vi "Auto Elevator Logic.vi"(8 "Has Trashcan?":bool, 10 "Elevator Sensors In":T7, 11 "Command":T3={"Command"=enum."Idle", "Manual Motor Out"=0.0, "Manual Eject Piston"=FALSE, "Mode"=enum."Manual", "Override Limits"=FALSE, "Manual Stabilizer"=FALSE, "Manual Finger"=FALSE, "Store Trashcan?"=FALSE, "Hold Low?"=FALSE, "Idle Mode"=enum."Load Can", "HP Load"=FALSE, "Unstick"=FALSE, "Raw Height Set"=0.0, "Force Store"=FALSE}) -> (0 "Trashcan Delta":i32, 1 "Tote Delta":i16, 2 "Elevator Actuators Out":T8, 3 "Auto Elevator Indicators":T1, 4 "Clear Stack Count":bool)   [LabVIEW 2014]
uses:
  Elevator Actuators.ctl
  Elevator Sensors.ctl
  Elevator Control Command.ctl
  Elevator Command.ctl
  Common Code/Elevator Mode.ctl
  Common Code/Elevator Idle Mode.ctl
  Common Code/Auto Elevator Indicators.ctl
  Common Code/Elevator State.ctl
  <vilib>/Rock Robotics/WPI/DriverStation/WPI_DriverStationRobotMode2.ctl
  Common Code/Change Detect Int.vi
  Robot Global Data.vi
panel:
  in  "# Totes Loading":i32
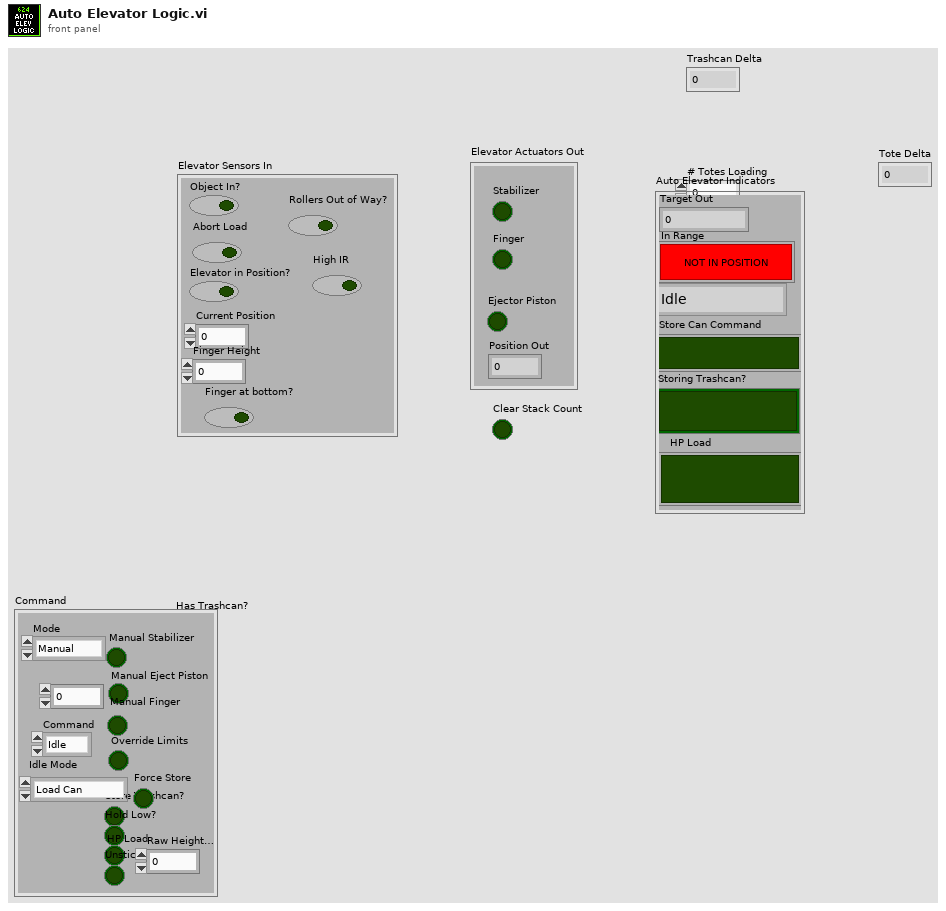
[diagram p1: front panel]
types:
  T1 = typedef "Auto Elevator Indicators.ctl" = cluster{"Target Out":dbl, "Storing Trashcan?":bool, "State":T2, "In Range":bool, "Store Can Command":bool, "HP Load":bool}
  T2 = typedef "Elevator State.ctl" = enum16{"Idle", "Goto Load Position", "Wait for Load", "Load Drop", "Load Lift", "Drop Stack", "Goto Eject Position", "Eject ", "Raise Trashcan", "Open Stabilizer", "Untip Drop", "Untip Wait", "Untip Lift", "Abort Load", "HP Load Wait", "HP Load Drop", "HP Load Lift", "HP Load Abort", "Close Stabilizer", "HP Load Unfinish", "HP Load Score", "HP Load Finish", "HP Goto Finish Down", "HP Goto Finish Up", "Full"}
  T3 = typedef "Elevator Control Command.ctl" = cluster{"Command":T4, "Manual Motor Out":dbl, "Manual Eject Piston":bool, "Mode":T5, "Override Limits":bool, "Manual Stabilizer":bool, "Manual Finger":bool, "Store Trashcan?":bool, "Hold Low?":bool, "Idle Mode":T6, "HP Load":bool, "Unstick":bool, "Raw Height Set":dbl, "Force Store":bool}
  T4 = typedef "Elevator Command.ctl" = enum16{"Idle", "Load 1", "Load 2", "Load 3", "Drop Stack", "Eject Stack", "Untip Trashcan", "Load Trashcan", "HP Load", "HP Score"}
  T5 = typedef "Elevator Mode.ctl" = enum16{"Manual", "Safe", "Auto"}
  T6 = typedef "Elevator Idle Mode.ctl" = enum16{"Load 1", "Load 2", "Load 3", "Load Can", "Untip Can", "Step Load", "Drop Stack", "Raw Height"}
  T7 = typedef "Elevator Sensors.ctl" = cluster{"Object In?":bool, "Elevator in Position?":bool, "Current Position":dbl, "Abort Load":bool, "Finger Height":dbl, "Finger at bottom?":bool, "Rollers Out of Way?":bool, "High IR":bool}
  T8 = typedef "Elevator Actuators.ctl" = cluster{"Ejector Piston":bool, "Finger":bool, "Stabilizer":bool, "Position Out":dbl}
  T9 = typedef "WPI_DriverStationRobotMode2.ctl" = enum16{"Autonomous Disabled", "Autonomous Enabled", "Teleop Disabled", "Teleop Enabled", "Disconnected", "Finish", "Test Disabled", "Test Enabled", "Emergency Stopped"}
  T10 = typedef "Dashboard Control Data.ctl" = cluster{"Cam Exposure":dbl, "Go to angle":dbl, "Steer PID Gains":cluster{"proportional gain (Kc)":dbl, "integral time (Ti, min)":dbl, "derivative time (Td, min)":dbl}, "Steer PID output Range":cluster{"output high":dbl, "output low":dbl}, "Pressure m \nValue":dbl, "Pressure b \nValue":dbl, "Roller Command Cluster ":T11, "Elevator":T12, "Encoder Control":T14, "Auton Settings":cluster{"Drive Dist Window Size":dbl}, "Drivetrain Settings":T15, "Lance":T16}
  T11 = typedef "Roller Control.ctl" = cluster{"Intake Speed":dbl, "Turn In Speed":dbl, "Unload Speed":dbl, "Turn Out Speed":dbl, "Ping Align Tolerance":dbl, "Tote Range Threshold":dbl, "Right Pot 0":dbl, "Pot Threshold":dbl, "Left Pot 0":dbl, "Right Pot Scale":dbl, "Left Pot Scale":dbl, "Min Elevator Height":dbl, "Eject Time":dbl, "Eject US Threshold":dbl, "Anti-Twitch Time":u32, "Ping Caring Threshold":dbl, "Pot Diff Threshold":dbl, "Pinch Sustain":u32, "Absorb Give Up Threshold":dbl, "Untip In Threshold":dbl, "Untip Grab Range":dbl, "Ultrasonic Hold Time":u32, "Landscape Absorb Time":u32, "Pot Use Wait Time":u32, "Can Turn Stop Range":dbl, "HP Load Speed":dbl, "Stick Multiplier":dbl}
  T12 = typedef "Elevator DB Control.ctl" = cluster{"PID Output Range":cluster{"output high":dbl, "output low":dbl}, "PID gains":cluster{"proportional gain (Kc)":dbl, "integral time (Ti, min)":dbl, "derivative time (Td, min)":dbl}, "Height Tolerance":sgl, " Encoder Constant":dbl, "Eject Time":sgl, "Zeroing Speed":sgl, "Presets":T13, "Ping Detect Threshold":sgl, "Trashcan Detect Threshold":sgl, "Zero Filter Time":dbl, "Stabilizer Open Time":dbl, "Zero Creep Speed":dbl, "Max Current":dbl, "Current Trip Time":dbl, "Abort Pitch":dbl, "Finger m":dbl, "Finger b":dbl, "Finger max ":dbl, "Finger Stabilizer":dbl, "Finger Store":dbl, "Finger Stop Store":dbl, "Stabilizer Close Time":dbl, "Finger min":dbl, "Unstick gain":dbl, "Full Detect Max":dbl}
  T13 = typedef "Elevator Presets.ctl" = cluster{"Pickup 2 w/ Tote":sgl, "Pickup 2 w/ Trashcan":sgl, "Pickup 3 w/ Tote":sgl, "Pickup 3 w/ Trashcan":sgl, "Bottom":sgl, "Pickup 1 w/ Tote":sgl, "Pickup Trashcan":sgl, "Pickup 1 w/ Trashcan":sgl, "Eject":sgl, "Hold Low":sgl, "Step add height":sgl, "Untip Lift":dbl, "Drop Stack":dbl, "HP Load Hold":dbl, "HP Load Drop":dbl, "HP Load Hold Can":dbl, "Store can max":dbl, "HP Drag Score":dbl, "HP Drag Finish":dbl, "Finger trashcan avoid":dbl, "Full":dbl}
  T14 = typedef "Encoder Control.ctl" = cluster{"Left Tick Constant":dbl, "Right Tick Constant":dbl, "Center Tick Constant":dbl, "Reset?":bool, "Y Dist":cluster{"PID gains":cluster{"proportional gain (Kc)":dbl, "integral time (Ti, min)":dbl, "derivative time (Td, min)":dbl}}, "X Dist":cluster{"PID gains":cluster{"proportional gain (Kc)":dbl, "integral time (Ti, min)":dbl, "derivative time (Td, min)":dbl}}, "Y Stop Thresh":dbl, "Y Stop Speed":dbl, "X Stop Thresh":dbl, "X Stop Speed":dbl}
  T15 = typedef "Drivetrain Settings.ctl" = cluster{"Gyro Tolerance":sgl, "Strafe Correct max steer":sgl, "Strafe Timer Wait":sgl, "Throttle Ramp (ms)":sgl, "Strafe Ramp (ms)":sgl, "Angular rate compensation":bool, "Throttle to Rate Scale":sgl, "Rate compensation gain":sgl, "Creep Steer":sgl, "Creep Throttle":sgl}
  T16 = typedef "Pike DB Controls.ctl" = cluster{"Down Speed":dbl, "Up Speed":dbl, "Max Down Time":dbl, "Max Up Time":dbl, "Current Limit":dbl}
  T17 = typedef "Roller Indicators.ctl" = cluster{"Rollers Closed?":bool, "Roller Mode":T18, "Auto Roller State":T19, "Tote Inside?":bool, "Intake State":T20, "Left Ping Dist":sgl, "Right Ping Dist":sgl, "Potentiometer Cluster":T21, "PING Decision":T20, "Left Arm Closed?":bool, "Portrait?":bool, "Right Arm Closed?":bool, "Left Out":sgl, "Right Out":sgl, "Left Current":sgl, "Right Current":sgl, "Tote Load Complete?":bool, "Untip Complete?":bool, "Untip State":T22, "Roller Safety Open":bool}
  T18 = typedef "Roller Mode Enum.ctl" = enum16{"Manual", "Safe", "Auto"}
  T19 = typedef "Auto Roller Commands.ctl" = enum16{"Drag Tote", "Grab Tote", "Idle", "Eject Tote", "Untip Can", "Grab Can"}
  T20 = typedef "Inner Roller States.ctl" = enum16{"Turn Tote Portrait", "Acquire Tote", "Absorb Tote", "Turn Tote Right", "Turn Tote Left", "Acquire Can", "Absorb Can", "Turn Can", "Hold Tote"}
  T21 = typedef "Pot Data.ctl" = cluster{"Left Pot Zero":sgl, "Right Pot Zero":sgl, "Left Potentiometer":sgl, "Right Potentiometer":sgl, "Left Pot Non Zero":sgl, "Right Pot Non Zero":sgl}
  T22 = typedef "Untip Can States.ctl" = enum16{"Release Can", "Catch Can", "Idle"}
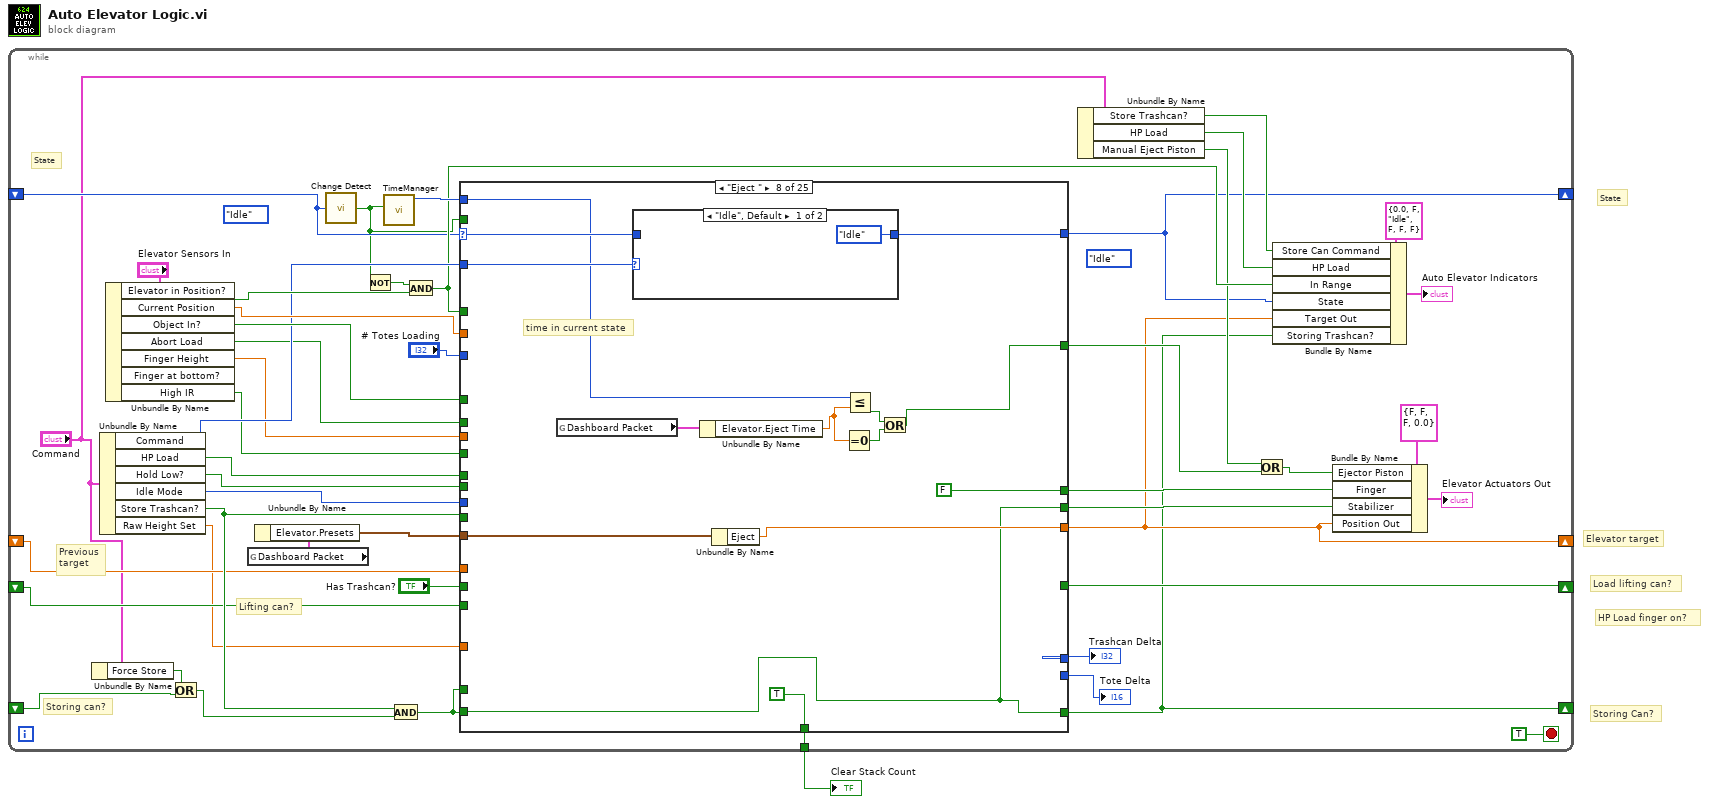
[diagram p0: block diagram]
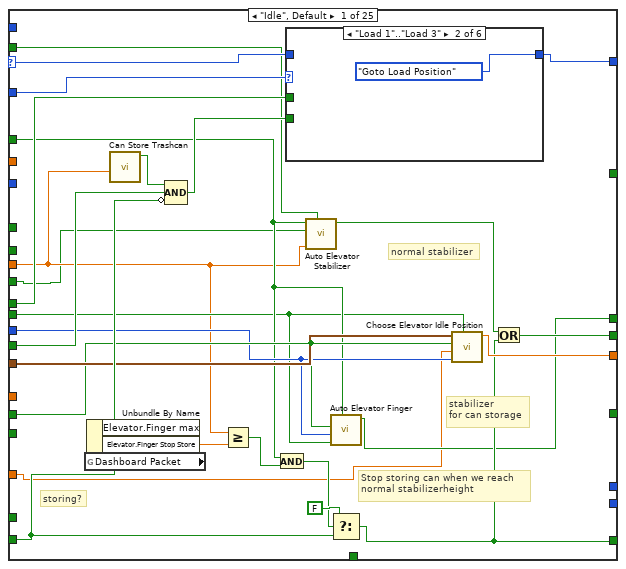
[diagram p2: hidden frame]
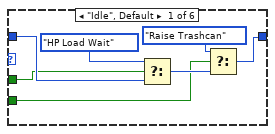
[diagram p3: hidden frame]
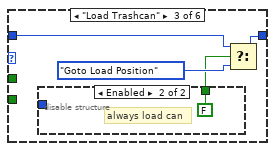
[diagram p4: hidden frame]
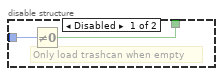
[diagram p5: hidden frame]
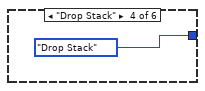
[diagram p6: hidden frame]
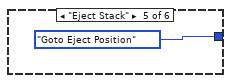
[diagram p7: hidden frame]
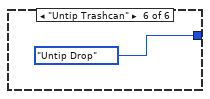
[diagram p8: hidden frame]
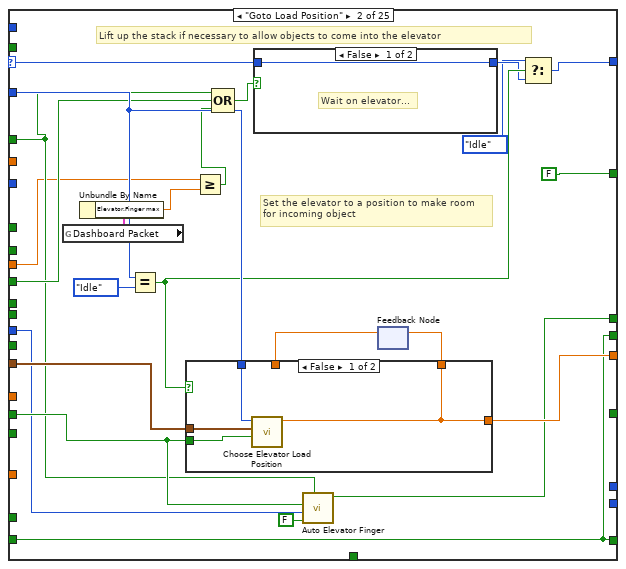
[diagram p9: hidden frame]
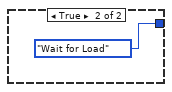
[diagram p11: hidden frame]
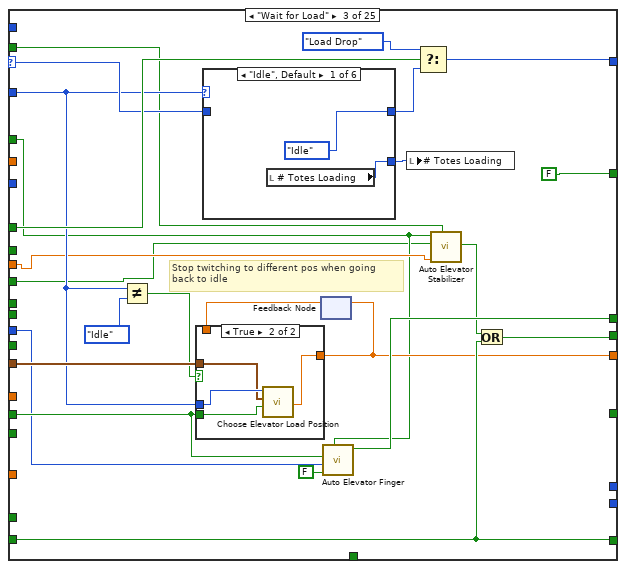
[diagram p12: hidden frame]
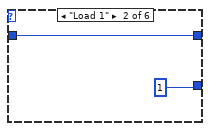
[diagram p13: hidden frame]
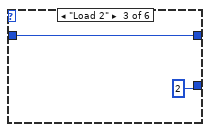
[diagram p14: hidden frame]
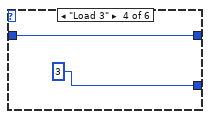
[diagram p15: hidden frame]
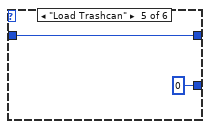
[diagram p16: hidden frame]
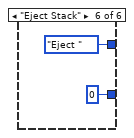
[diagram p17: hidden frame]
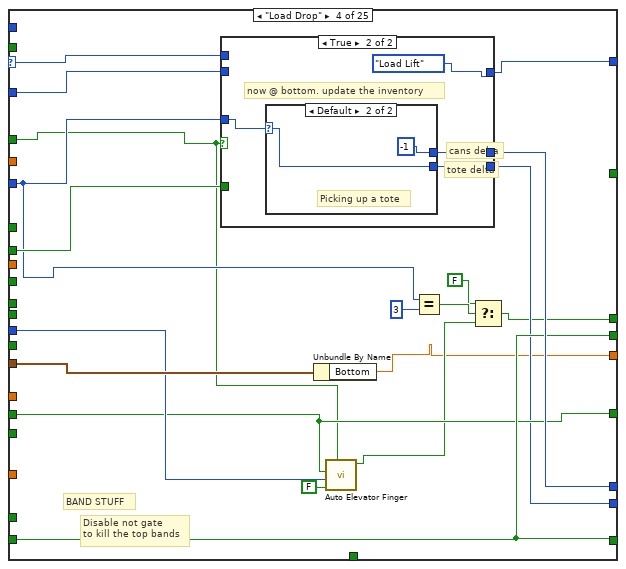
[diagram p19: hidden frame]
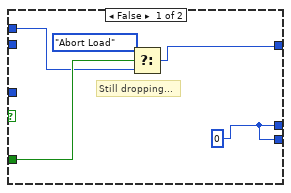
[diagram p20: hidden frame]
diagram:
  # "State"
  # "Storing Can?"
  # "HP Load finger on?"
  # "Load lifting can?"
  # "Elevator target"
  n1 = while {
    tunnel: [w39] -> w1
    shift-right: [w18] -> _
    shift-left: _ -> [w17]
    shift-right: [w16] -> _
    shift-left: _ -> [w15]
    shift-right: [w14] -> _
    shift-left: _ -> [w4]
    shift-right: [w8] -> _
    shift-left: _ -> [w13]
    stop <- TRUE stop-if-true
    (unwired) Elevator_State."Idle" ("f")
    (unwired) Elevator_State."Idle" ("f")
    # "Storing can?"
    # "State"
    # "Lifting can?"
    # "Previous\ntarget"
    n2 = Unbundle By Name("Command") -> ("Force Store"=w3:bool)
    n3 = Unbundle By Name("Command") -> ("Command"=w36:T4, "HP Load"=w28:bool, "Hold Low?"=w31:bool, "Idle Mode"=w30:T6, "Store Trashcan?"=w35:bool, "Raw Height Set"=w6:dbl)
    n4 = Unbundle By Name("Elevator Sensors In") -> ("Elevator in Position?"=w47:bool, "Current Position"=w45:dbl, "Object In?"=w46:bool, "Abort Load"=w29:bool, "Finger Height"=w22:dbl, "High IR"=w7:bool)  [unwired: 1 out]
    n5 = Or(x=w3, y=w4) -> (x .or. y?=w2:bool)
    n6 = global read "Robot Global Data.vi" "Dashboard Packet"() -> (w12:T10)
    n7 = Unbundle By Name(w12) -> ("Elevator.Presets"=w38:T13)
    n8 = call-poly "Change Detect.vi"("In"=w13) -> ("Changed?"=w9:bool)
    n9 = Not(x=w9) -> (.not. x?=w49:bool)
    n10 = call "TimeManager.vi"("Reset?"=w9) -> ("Time Since Reset"=w37:u32)  [unwired: 9 in, 1 out]
    n11 = And(x=w35, y=w2) -> (x .and. y?=w10:bool)
    n12 = And(x=w49, y=w47) -> (x .and. y?=w32:bool)
    n13 = case shown="\"Eject \"" w13 {
      selector: w13 -> [w59 w116 w146 w182 w231 w254 w271 w290 w304 w332 w351 w366 w376 w398 w410 w460 w477 w487 w501 w507 w516 w528 w540 w556 w570]
      tunnel: [_ FALSE ("Ejector Piston") FALSE ("Ejector Piston") _ FALSE ("Ejector Piston") FALSE ("Ejector Piston") FALSE ("Ejector Piston") w283 FALSE ("Ejector Piston") FALSE ("Ejector Piston") w355 w369 w379 _ _ _ _ _ _ _ _ _ _ _ _] -> w25
      tunnel: w38 -> [w65 w115 w143 w185 w218 w257 w275 w293 _ w331 w357 w371 w381 w390 w409 w462 w464 w493 _ _ w522 _ w545 w567 w577]
      tunnel: [w75 w118 w139 w168 w228 w256 w274 w292 w299 w323 w356 w370 w380 w396 w419 w461 w463 w481 w496 w513 w521 w525 w544 w566 w576] -> w18
      tunnel: w45 -> [_ _ _ _ w206 _ _ _ _ w322 _ _ _ _ w408 _ _ _ _ _ _ w525 _ _ _]
      tunnel: w46 -> [_ _ w148 _ _ w253 _ _ _ _ _ _ _ _ _ _ _ _ _ _ _ _ _ _ _]
      tunnel: w36 -> [w76 w112 w137 w183 w235 w255 w272 w291 w312 w336 w354 w364 w374 w394 w412 _ _ w492 _ _ w518 w530 w541 w557 w572]
      tunnel: w32 -> [w56 w100 w130 w167 w204 w248 w267 _ _ w329 w348 _ _ w386 _ w459 w475 w489 _ _ _ _ w539 w561 _]
      tunnel: "# Totes Loading" -> [_ _ _ w175 _ _ _ _ _ _ _ _ _ _ _ _ _ _ _ _ _ _ _ _ _]
      tunnel: "Has Trashcan?" -> [w62 w105 w132 w178 w226 w250 w269 _ _ _ _ _ _ w388 w405 w451 _ w478 _ _ _ _ _ _ _]
      tunnel: [_ _ _ w184 _ _ _ _ _ w341 _ _ _ _ _ _ -1 ("f") _ _ _ _ _ _ _ _] -> w41
      tunnel: [w57 w113 w140 w170 w224 w245 w270 FALSE TRUE TRUE w355 w369 w379 w403 w406 w450 TRUE ("Boolean") w479 TRUE ("Boolean") TRUE ("Boolean") w520 w527 TRUE ("Boolean") TRUE ("Boolean") TRUE ("Boolean")] -> w21
      tunnel: [w72 w114 w141 w181 w220 w245 w264 w281 FALSE FALSE w355 w369 w379 w402 w413 w452 w469 FALSE TRUE ("Close stabilizer") FALSE ("Boolean") w520 w527 FALSE ("Boolean") w548 TRUE ("t")] -> w20
      tunnel: [_ _ _ _ _ w252 _ TRUE _ _ _ _ _ _ _ _ _ _ _ _ _ _ _ _ _] -> w39
      tunnel: w37 -> [_ _ _ _ _ _ _ w287 w307 _ _ _ _ _ _ _ _ _ w504 w508 _ _ _ _ _]
      tunnel: [w71 w114 w142 w181 w222 FALSE w264 w281 FALSE ("x >= y?") w327 FALSE ("x >= y?") FALSE ("x >= y?") FALSE ("x >= y?") w401 w413 w452 w469 FALSE ("x >= y?") TRUE ("x >= y?") FALSE ("x >= y?") FALSE ("t") FALSE ("t") FALSE ("t") w548 FALSE ("t")] -> w14
      tunnel: w10 -> [w69 w114 w142 w181 w222 _ w264 w281 _ _ _ _ _ w401 w415 w452 w471 _ _ _ _ _ _ w554 _]
      tunnel: w35 -> [w70 _ _ _ _ _ _ _ w313 w337 _ _ _ _ _ _ _ _ _ _ _ _ _ _ _]
      tunnel: w31 -> [w55 _ _ _ w229 w247 _ _ _ _ _ _ _ _ _ _ _ _ _ _ _ _ _ _ _]
      tunnel: w30 -> [w61 w104 w131 w179 w227 _ w268 _ _ _ _ _ _ w387 _ _ _ _ _ _ _ _ _ _ _]
      tunnel: w29 -> [_ _ _ w180 _ _ _ _ _ _ _ _ _ _ _ w456 _ _ _ _ _ _ _ _ _]
      tunnel: w28 -> [w58 _ _ _ _ _ _ _ _ _ _ _ _ _ w411 _ _ _ _ _ _ _ _ _ _]
      tunnel: w22 -> [w53 w98 w133 _ w214 _ _ _ w301 w321 _ _ _ w389 w404 _ w473 _ _ _ _ _ _ w553 _]
      tunnel: [_ _ _ w178 w216 _ _ _ _ _ _ _ _ _ _ _ _ _ _ _ _ _ _ _ _] -> w16
      tunnel: w17 -> [_ _ _ _ _ _ _ _ w299 _ _ _ _ _ _ _ _ _ w496 w513 _ _ _ _ _]
      tunnel: w15 -> [_ _ _ _ w216 _ _ _ _ _ _ _ _ _ _ _ _ _ _ _ _ _ _ _ _]
      tunnel: [_ _ _ w177 _ _ _ _ _ _ _ _ _ _ _ w449 _ _ _ _ _ _ _ _ _] -> w11
      tunnel: w10 -> [_ _ _ _ _ _ _ _ _ _ _ _ _ _ _ _ _ _ _ _ _ _ _ _ _]
      tunnel: w9 -> [w51 _ w126 _ _ _ _ _ _ _ _ _ _ w382 _ _ _ _ _ _ _ _ _ _ _]
      tunnel: [w54 w102 w128 w169 w208 w246 w265 w282 w297 w318 w345 w358 w372 w384 w407 w448 w465 w480 w494 w505 w517 w529 w536 w559 w571] -> w8
      tunnel: w7 -> [w52 w101 w127 _ w211 _ _ _ _ _ _ _ _ w383 _ _ _ _ _ _ _ _ _ _ _]
      tunnel: w6 -> [w50 _ _ _ w213 _ _ _ _ _ _ _ _ _ _ _ _ _ _ _ _ _ _ _ _]
      frame "Idle", Default {
        # "storing?"
        # "stabilizer\nfor can storage"
        # "normal stabilizer"
        # "Stop storing can when we reach\nnormal stabilizerheight"
        n14 = global read "Robot Global Data.vi" "Dashboard Packet"() -> (w66:T10)
        n15 = Unbundle By Name(w66) -> ("Elevator.Finger Stop Store"=w68:dbl)  [unwired: 1 out]
        n16 = call "Can Store Trashcan.vi"("Finger height"=w53) -> ("Boolean"=w67:bool)  [unwired: 10 in]
        n17 = Compound Arithmetic op=AND(w67, w70, invert w69) -> (w60:bool)
        n18 = Greater Or Equal?(x=w53, y=w68) -> (x >= y?=w64:bool)
        n19 = And(x=w56, y=w64) -> (x .and. y?=w63:bool)
        n20 = case shown="\"Load 1\"..\"Load 3\"" w76 {
          tunnel: w59 -> [w79 _ w87 _ _ _]
          tunnel: [w83 Elevator_State."Goto Load Position" ("Enum") w86 Elevator_State."Drop Stack" ("Enum") Elevator_State."Goto Eject Position" ("Enum") Elevator_State."Untip Drop" ("Enum")] -> w54
          tunnel: w60 -> [w78 _ _ _ _ _]
          tunnel: w58 -> [w77 _ _ _ _ _]
          frame "Idle", Default {
            n21 = Select(t=Elevator_State."HP Load Wait", s=w77, f=w79) -> (s? t:f=w82:T2)
            n22 = Select(t=Elevator_State."Raise Trashcan", s=w78, f=w82) -> (s? t:f=w83:T2)
          }
          frame "Load 1".."Load 3" {
          }
          frame "Load Trashcan" {
            n23 = disable-structure shown="Enabled" {
              disable-tunnel: _ -> [w90 _]
              disable-tunnel: [w89 FALSE] -> w85
              frame Disabled {
                # "Only load trashcan when empty"
                n24 = Not Equal To 0?(x=w90) -> (x != 0?=w89:bool)
              }
              frame Enabled {
                # "always load can"
              }
            }
            n25 = Select(t=w87, s=w85, f=Elevator_State."Goto Load Position" ("Enum")) -> (s? t:f=w86:T2)
          }
          frame "Drop Stack" {
          }
          frame "Eject Stack" {
          }
          frame "Untip Trashcan" {
          }
        }
        n26 = call "Auto Elevator Stabilizer.vi"("State  Change?"=w51, "Finger Height"=w53, "High IR"=w52, "Elevator in position?"=w56) -> ("Close stabilizer"=w73:bool)  [unwired: 7 in]
        n27 = call "Auto Elevator Finger.vi"("Elevator in Position"=w56, "Hold Low"=w55, "Idle Mode"=w61, "Has Trashcan"=w62) -> ("Finger On?"=w57:bool)  [unwired: 7 in]
        n28 = Select(t=FALSE ("x >= y?"), s=w63, f=w69) -> (s? t:f=w71:bool)
        n29 = call "Choose Elevator Idle Position.vi"("Hold Low?"=w55, "Idle Mode"=w61, "Raw Height Set"=w50, "Has Trashcan?"=w62, "Presets"=w65) -> ("Pos Out"=w75:sgl)  [unwired: 6 in]
        n30 = Or(x=w73, y=w71) -> (x .or. y?=w72:bool)
      }
      frame "Goto Load Position" {
        # "Set the elevator to a position to make room\nfor incoming object"
        # "Lift up the stack if necessary to allow objects to come into the elevator"
        n31 = global read "Robot Global Data.vi" "Dashboard Packet"() -> (w97:T10)
        n32 = Unbundle By Name(w97) -> ("Elevator.Finger max"=w96:dbl)
        n33 = Equal?(x=w112, y=Elevator_Command."Idle") -> (x = y?=w108:bool)
        n34 = Greater Or Equal?(x=w98, y=w96) -> (x >= y?=w95:bool)
        n35 = Compound Arithmetic op=OR(w100, w101, w95) -> (w99:bool)
        n36 = case shown="False" w99 {
          tunnel: w116 -> [w124 _]
          tunnel: [w124 Elevator_State."Wait for Load" ("Enum")] -> w107
          frame False {
            # "Wait on elevator..."
          }
          frame True {
          }
        }
        n37 = call "Auto Elevator Finger.vi"("Elevator in Position"=w100, "Hold Low"=FALSE, "Idle Mode"=w104, "Has Trashcan"=w105) -> ("Finger On?"=w113:bool)  [unwired: 7 in]
        n38 = feedback #1() -> (w110:dbl)  [unwired: 1 in]
        n39 = case shown="False" w108 {
          tunnel: w112 -> [w122 _]
          tunnel: [w120 w123] -> w118
          tunnel: w105 -> [w121 _]
          tunnel: w115 -> [w119 _]
          tunnel: w110 -> [_ w123]
          tunnel: [w120 w123] -> w109
          frame False {
            n40 = call "Choose Elevator Load Position.vi"("Have Trashcan?"=w121, "Presets"=w119, "Command"=w122) -> ("Elevator Position"=w120:dbl)  [unwired: 8 in]
          }
          frame True {
            # "Keep going even when button\nnot still pressed"
          }
        }
        n41 = feedback-in #1(w109) -> ()
        n42 = Select(t=Elevator_State."Idle", s=w108, f=w107) -> (s? t:f=w102:T2)
      }
      frame "Wait for Load" {
        # "Stop twitching to different pos when going \nback to idle"
        n43 = Not Equal?(x=w137, y=Elevator_Command."Idle") -> (x != y?=w135:bool)
        n44 = case shown="\"Idle\", Default" w137 {
          tunnel: w146 -> [_ w153 w155 w157 w158 _]
          tunnel: [Elevator_State."Idle" ("Enum") w153 w155 w157 w158 Elevator_State."Eject " ("Enum")] -> w145
          tunnel: [w151 1 2 3 0 ("# Totes Loading") 0 ("# Totes Loading")] -> w144
          frame "Idle", Default {
            n45 = local read "# Totes Loading"() -> (w151:i32)
          }
          frame "Load 1" {
          }
          frame "Load 2" {
          }
          frame "Load 3" {
          }
          frame "Load Trashcan" {
          }
          frame "Eject Stack" {
          }
        }
        n46 = feedback #2() -> (w138:dbl)  [unwired: 1 in]
        n47 = case shown="True" w135 {
          tunnel: w137 -> [_ w166]
          tunnel: w143 -> [_ w164]
          tunnel: [w162 w165] -> w139
          tunnel: w138 -> [w162 _]
          tunnel: w132 -> [_ w163]
          frame False {
          }
          frame True {
            n48 = call "Choose Elevator Load Position.vi"("Have Trashcan?"=w163, "Presets"=w164, "Command"=w166) -> ("Elevator Position"=w165:dbl)  [unwired: 8 in]
          }
        }
        n49 = feedback-in #2(w139) -> ()
        n50 = call "Auto Elevator Finger.vi"("Elevator in Position"=w130, "Hold Low"=FALSE, "Idle Mode"=w131, "Has Trashcan"=w132) -> ("Finger On?"=w140:bool)  [unwired: 7 in]
        n51 = local write "# Totes Loading"(w144) -> ()
        n52 = Select(t=Elevator_State."Load Drop" ("Enum"), s=w148, f=w145) -> (s? t:f=w128:T2)
        n53 = call "Auto Elevator Stabilizer.vi"("State  Change?"=w126, "Finger Height"=w133, "High IR"=w127, "Elevator in position?"=w130) -> ("Close stabilizer"=w134:bool)  [unwired: 7 in]
        n54 = Or(x=w134, y=w142) -> (x .or. y?=w141:bool)
      }
      frame "Load Drop" {
        # "Disable not gate\nto kill the top bands"
        # "BAND STUFF"
        # "tote delta"
        # "cans delta"
        n55 = case shown="True" w167 {
          tunnel: w183 -> [_ _]
          tunnel: w175 -> [_ w191]
          tunnel: [w190 w194] -> w184
          tunnel: [w190 w193] -> w177
          tunnel: [w186 Elevator_State."Load Lift" ("Enum")] -> w169
          tunnel: w182 -> [w188 _]
          tunnel: w180 -> [w189 _]
          frame False {
            w190 = 0
            # "Still dropping..."
            n56 = Select(t=Elevator_State."Abort Load", s=w189, f=w188) -> (s? t:f=w186:T2)
          }
          frame True {
            # "now @ bottom. update the inventory"
            n57 = case shown="Default" w191 {
              selector: w191 -> [_ w197]
              tunnel: [1 -1] -> w194
              tunnel: [-999 ("# Totes Loading") w197] -> w193
              frame 0 {
                # "clear \ntote count"
                # "Picking up a can"
              }
              frame Default {
                # "Picking up a tote"
              }
            }
          }
        }
        n58 = Unbundle By Name(w185) -> ("Bottom"=w168:sgl)
        n59 = call "Auto Elevator Finger.vi"("Elevator in Position"=w167, "Hold Low"=FALSE, "Idle Mode"=w179, "Has Trashcan"=w178) -> ("Finger On?"=w171:bool)  [unwired: 7 in]
        n60 = Equal?(x=w175, y=3) -> (x = y?=w173:bool)
        n61 = Select(t=FALSE, s=w173, f=w171) -> (s? t:f=w170:bool)
      }
      frame "Load Lift" {
        # "We hit a limit\non the way up"
        # "Allow Drop Stack to\nabort Load Lift"
        n62 = call "Auto Elevator Finger.vi"("Elevator in Position"=w204, "Hold Low"=FALSE, "Idle Mode"=w227, "Has Trashcan"=w226) -> ("Finger On?"=w225:bool)  [unwired: 7 in]
        n63 = global read "Robot Global Data.vi" "Dashboard Packet"() -> (w219:T10)
        n64 = Unbundle By Name(w219) -> ("Elevator.Full Detect Max"=w205:dbl, "Elevator.Finger max"=w217:dbl, "Elevator.Finger Stop Store"=w223:dbl)
        n65 = case shown="True" w216 {
          tunnel: w225 -> [w238 w243]
          tunnel: [w238 w244] -> w224
          tunnel: w218 -> [_ w241]
          tunnel: w206 -> [_ w239]
          frame False {
            # "Didn't just have a can"
          }
          frame True {
            n66 = Unbundle By Name(w241) -> ("Finger trashcan avoid"=w240:dbl)
            n67 = Greater Or Equal?(x=w239, y=w240) -> (x >= y?=w242:bool)
            n68 = And(x=w243, y=w242) -> (x .and. y?=w244:bool)
          }
        }
        n69 = Equal?(x=Elevator_Command."Drop Stack", y=w235) -> (x = y?=w233:bool)
        n70 = Select(t=Elevator_State."Drop Stack", s=w233, f=w231) -> (s? t:f=w230:T2)
        n71 = Greater Or Equal?(x=w214, y=w217) -> (x >= y?=w212:bool)
        n72 = call "Choose Elevator Idle Position.vi"("Hold Low?"=w229, "Idle Mode"=w227, "Raw Height Set"=w213, "Has Trashcan?"=w226, "Presets"=w218) -> ("Pos Out"=w228:sgl)  [unwired: 6 in]
        n73 = Or(x=w212, y=w211) -> (x .or. y?=w201:bool)
        n74 = Less Or Equal?(x=w206, y=w205) -> (x <= y?=w207:bool)
        n75 = And(x=w201, y=w207) -> (x .and. y?=w203:bool)
        n76 = Not(x=w203) -> (.not. x?=w202:bool)
        n77 = And(x=w201, y=w202) -> (x .and. y?=w200:bool)
        n78 = Or(x=w204, y=w200) -> (x .or. y?=w199:bool)
        n79 = Select(t=Elevator_State."Idle", s=w199, f=w230) -> (s? t:f=w209:T2)
        n80 = Less?(x=w214, y=w223) -> (x < y?=w221:bool)
        n81 = And(x=w221, y=w222) -> (x .and. y?=w220:bool)
        n82 = Select(t=Elevator_State."Full", s=w203, f=w209) -> (s? t:f=w208:T2)
      }
      frame "Drop Stack" {
        w245 = FALSE
        # "override idle\nmode stuff for\nthis case"
        n83 = case shown="Default" w255 {
          tunnel: w254 -> [_ w263]
          tunnel: [Elevator_State."Idle" ("Enum") w263] -> w246
          tunnel: w253 -> [w260 _]
          tunnel: w250 -> [_ _]
          tunnel: [w259 FALSE] -> w252
          frame Default {
            # "Done dropping. See \nif stuff is gone"
            n84 = Not(x=w260) -> (.not. x?=w259:bool)
          }
          frame "Drop Stack" {
            # "Still dropping..?"
          }
        }
        n85 = Unbundle By Name(w257) -> ("Drop Stack"=w256:dbl)
        n86 = call "Auto Elevator Finger.vi"("Elevator in Position"=w248, "Hold Low"=w247, "Idle Mode"=Elevator_Idle_Mode."Load 1", "Has Trashcan"=w250) -> ()  [unwired: 7 in, 1 out]
      }
      frame "Goto Eject Position" {
        n87 = Unbundle By Name(w275) -> ("Eject"=w274:sgl)
        n88 = case shown="\"Eject Stack\"" w272 {
          tunnel: w271 -> [_ w279]
          tunnel: [Elevator_State."Idle" ("Enum") w277] -> w265
          tunnel: w267 -> [_ w280]
          frame "Idle", Default {
          }
          frame "Eject Stack" {
            n89 = Select(t=Elevator_State."Eject ", s=w280, f=w279) -> (s? t:f=w277:T2)
          }
        }
        n90 = call "Auto Elevator Finger.vi"("Elevator in Position"=w267, "Hold Low"=FALSE, "Idle Mode"=w268, "Has Trashcan"=w269) -> ("Finger On?"=w270:bool)  [unwired: 7 in]
      }
      frame "Eject " {
        # "time in current state"
        n91 = global read "Robot Global Data.vi" "Dashboard Packet"() -> (w288:T10)
        n92 = case shown="\"Idle\", Default" w291 {
          tunnel: w290 -> [_ w296]
          tunnel: [Elevator_State."Idle" ("Enum") w296] -> w282
          frame "Idle", Default {
          }
          frame "Eject Stack" {
          }
        }
        n93 = Unbundle By Name(w288) -> ("Elevator.Eject Time"=w286:sgl)
        n94 = Unbundle By Name(w293) -> ("Eject"=w292:sgl)
        n95 = Equal To 0?(x=w286) -> (x = 0?=w284:bool)
        n96 = Less Or Equal?(x=w287, y=w286) -> (x <= y?=w285:bool)
        n97 = Or(x=w285, y=w284) -> (x .or. y?=w283:bool)
      }
      frame "Open Stabilizer" {
        # "Hold current position while\nwaiting for stabilizer to open"
        # "Remove can from count when stored"
        n98 = global read "Robot Global Data.vi" "Dashboard Packet"() -> (w308:T10)
        n99 = Unbundle By Name(w308) -> ("Elevator.Stabilizer Open Time"=w306:dbl)
        n100 = Greater Or Equal?(x=w307, y=w306) -> (x >= y?=w305:bool)
        n101 = Select(t=Elevator_State."Raise Trashcan", s=w305, f=w304) -> (s? t:f=w303:T2)
        n102 = Equal?(x=w312, y=Elevator_Command."Idle") -> (x = y?=w310:bool)
        n103 = call "Can Store Trashcan.vi"("Finger height"=w301) -> ("Boolean"=w314:bool)  [unwired: 10 in]
        n104 = Compound Arithmetic op=AND(w314, w313, w310) -> (w309:bool)
        n105 = Select(t=w303, s=w309, f=Elevator_State."Idle") -> (s? t:f=w297:T2)
      }
      frame "Raise Trashcan" {
        # "hold @ current pos\nif finger @ right \nheight"
        # "Raising trashcan for can storage"
        # "Remove can from count when stored"
        n106 = global read "Robot Global Data.vi" "Dashboard Packet"() -> (w320:T10)
        n107 = Unbundle By Name(w331) -> ("Store can max"=w324:dbl)
        n108 = Unbundle By Name(w320) -> ("Elevator.Finger Store"=w330:dbl)
        n109 = Equal?(x=w336, y=Elevator_Command."Idle") -> (x = y?=w334:bool)
        n110 = call "Can Store Trashcan.vi"("Finger height"=w321) -> ("Boolean"=w338:bool)  [unwired: 10 in]
        n111 = Greater Or Equal?(x=w321, y=w330) -> (x >= y?=w325:bool)
        n112 = Compound Arithmetic op=AND(w338, w337, w334) -> (w333:bool)
        n113 = Or(x=w329, y=w325) -> (x .or. y?=w327:bool)
        n114 = Select(t=w332, s=w333, f=Elevator_State."Idle" ("t")) -> (s? t:f=w328:T2)
        n115 = Select(t=w322, s=w325, f=w324) -> (s? t:f=w323:dbl)
        n116 = Select(t=Elevator_State."Close Stabilizer", s=w327, f=w328) -> (s? t:f=w318:T2)
        n117 = Select(t=-1 ("lower limit"), s=w327, f=0) -> (s? t:f=w341:i32)
      }
      frame "Untip Drop" {
        w355 = FALSE
        n118 = Equal?(x=w354, y=Elevator_Command."Untip Trashcan") -> (x = y?=w352:bool)
        n119 = Unbundle By Name(w357) -> ("Bottom"=w356:sgl)
        n120 = Select(t=w351, s=w352, f=Elevator_State."Idle") -> (s? t:f=w349:T2)
        n121 = Select(t=Elevator_State."Untip Wait", s=w348, f=w349) -> (s? t:f=w345:T2)
      }
      frame "Untip Wait" {
        w369 = FALSE
        n122 = Equal?(x=w364, y=Elevator_Command."Untip Trashcan") -> (x = y?=w368:bool)
        n123 = global read "Robot Global Data.vi" "Roller State Indicators"() -> (w360:T17)
        n124 = Unbundle By Name(w371) -> ("Bottom"=w370:sgl)
        n125 = Select(t=w366, s=w368, f=Elevator_State."Idle") -> (s? t:f=w363:T2)
        n126 = Unbundle By Name(w360) -> ("Untip Complete?"=w359:bool)
        n127 = Select(t=Elevator_State."Untip Lift", s=w359, f=w363) -> (s? t:f=w358:T2)
      }
      frame "Untip Lift" {
        w379 = FALSE
        n128 = Equal?(x=w374, y=Elevator_Command."Load Trashcan") -> (x = y?=w378:bool)
        n129 = Unbundle By Name(w381) -> ("Untip Lift"=w380:dbl)
        n130 = Select(t=Elevator_State."Idle" ("f"), s=w378, f=w376) -> (s? t:f=w372:T2)
      }
      frame "Abort Load" {
        # "Stay away until command goes back to idle"
        # "Run away! Stop breaking the robot! Back to the up position!"
        n131 = Equal?(x=Elevator_Command."Drop Stack" ("y"), y=w394) -> (x = y?=w392:bool)
        n132 = Equal?(x=w394, y=Elevator_Command."Idle") -> (x = y?=w393:bool)
        n133 = Or(x=w393, y=w392) -> (x .or. y?=w391:bool)
        n134 = call "Auto Elevator Stabilizer.vi"("State  Change?"=w382, "Finger Height"=w389, "High IR"=w383, "Elevator in position?"=w386) -> ("Close stabilizer"=w400:bool)  [unwired: 7 in]
        n135 = Select(t=Elevator_State."Idle", s=w391, f=w398) -> (s? t:f=w384:T2)
        n136 = call "Choose Elevator Load Position.vi"("Have Trashcan?"=w388, "Presets"=w390, "Command"=w394) -> ("Elevator Position"=w396:dbl)  [unwired: 8 in]
        n137 = call "Auto Elevator Finger.vi"("Elevator in Position"=w386, "Hold Low"=FALSE, "Idle Mode"=w387, "Has Trashcan"=w388) -> ("Finger On?"=w403:bool)  [unwired: 7 in]
        n138 = Or(x=w400, y=w401) -> (x .or. y?=w402:bool)
      }
      frame "HP Load Wait" {
        n139 = case shown="\"Load Trashcan\"" w412 {
          tunnel: w411 -> [w426 _ _ _]
          tunnel: w410 -> [w433 _ _ _]
          tunnel: w409 -> [_ _ w446 _]
          tunnel: w408 -> [_ _ w444 _]
          tunnel: [w422 Elevator_State."HP Load Drop" ("t") w435 Elevator_State."HP Load Score" ("f")] -> w407
          tunnel: w404 -> [_ _ w442 _]
          frame "Idle", Default {
            # "Stay in HP if robot is disabled"
            # "(Going to Idle will unset the\nHP mode toggle inside Teleop\nElevator Control)"
            # "Exit HP Mode?"
            n140 = call <vilib>:"WPI_DriverStationGetModeAndStatus.vi"() -> ("Robot Mode"=w430:T9)  [unwired: 10 in, 1 out]
            n141 = Equal?(x=w430, y=WPI_DriverStationRobotMode2."Autonomous Enabled") -> (x = y?=w428:bool)
            n142 = Equal?(x=w430, y=WPI_DriverStationRobotMode2."Teleop Enabled") -> (x = y?=w427:bool)
            n143 = Or(x=w428, y=w427) -> (x .or. y?=w423:bool)
            n144 = Not(x=w423) -> (.not. x?=w424:bool)
            n145 = Or(x=w426, y=w424) -> (x .or. y?=w425:bool)
            n146 = Select(t=w433, s=w425, f=Elevator_State."Idle") -> (s? t:f=w422:T2)
          }
          frame "Load 1" {
            # "HP Load a tote"
          }
          frame "Load Trashcan" {
            # "nope"
            # "yes"
            # "Check if that's\nhigh enough\nfor stabilizer"
            # "So subtract that to\npredict finger height at\nDrag Finish"
            # "Elevator will go down\nthis much to get to Drag\nFinish setpoint"
            # "X button. Prepare to\nscore stack. The elevator may need to go\nUP to get the can to be storable"
            n147 = Unbundle By Name(w446) -> ("HP Drag Finish"=w445:dbl)
            n148 = Subtract(x=w444, y=w445) -> (x-y=w443:dbl)
            n149 = global read "Robot Global Data.vi" "Dashboard Packet"() -> (w440:T10)
            n150 = Unbundle By Name(w440) -> ("Elevator.Finger Store"=w439:dbl)
            n151 = Subtract(x=w442, y=w443) -> (x-y=w441:dbl)
            n152 = Greater Or Equal?(x=w441, y=w439) -> (x >= y?=w438:bool)
            n153 = Select(t=Elevator_State."HP Goto Finish Down" ("f"), s=w438, f=Elevator_State."HP Goto Finish Up") -> (s? t:f=w435:T2)
          }
          frame "Load 3", "Drop Stack" {
            # "Manipulator drop stack override. \nProbably not useful"
          }
        }
        n154 = Unbundle By Name(w409) -> ("HP Load Hold Can"=w421:dbl, "HP Load Hold"=w420:dbl)
        n155 = global read "Robot Global Data.vi" "Dashboard Packet"() -> (w418:T10)
        n156 = Unbundle By Name(w418) -> ("Elevator.Finger Stop Store"=w417:dbl)
        n157 = Greater Or Equal?(x=w404, y=w417) -> (x >= y?=w416:bool)
        n158 = Select(t=w421, s=w405, f=w420) -> (s? t:f=w419:dbl)
        n159 = Select(t=FALSE, s=w416, f=w415) -> (s? t:f=w413:bool)
        n160 = Not(x=w405) -> (.not. x?=w406:bool)
      }
      frame "HP Load Drop" {
        # "Put finger off\nwhen we are holding a can"
        n161 = Unbundle By Name(w462) -> ("HP Load Drop"=w461:dbl)
        n162 = Select(t=Elevator_State."HP Load Lift", s=w459, f=w460) -> (s? t:f=w455:T2)
        n163 = Select(t=Elevator_State."HP Load Abort", s=w456, f=w455) -> (s? t:f=w448:T2)
        n164 = Select(t=1, s=w459, f=0) -> (s? t:f=w449:i32)
        n165 = Not(x=w451) -> (.not. x?=w450:bool)
      }
      frame "HP Load Lift" {
        n166 = global read "Robot Global Data.vi" "Dashboard Packet"() -> (w467:T10)
        n167 = Unbundle By Name(w467) -> ("Elevator.Finger Stop Store"=w466:dbl)
        n168 = Greater Or Equal?(x=w473, y=w466) -> (x >= y?=w472:bool)
        n169 = Unbundle By Name(w464) -> ("HP Load Hold"=w463:dbl)
        n170 = Select(t=Elevator_State."HP Load Wait", s=w475, f=w477) -> (s? t:f=w465:T2)
        n171 = Select(t=FALSE ("x >= y?"), s=w472, f=w471) -> (s? t:f=w469:bool)
      }
      frame "HP Load Abort" {
        n172 = Equal?(x=w492, y=Elevator_Command."Idle") -> (x = y?=w490:bool)
        n173 = And(x=w490, y=w489) -> (x .and. y?=w488:bool)
        n174 = Unbundle By Name(w493) -> ("HP Load Hold Can"=w483:dbl, "HP Load Hold"=w482:dbl)
        n175 = Select(t=Elevator_State."HP Load Wait", s=w488, f=w487) -> (s? t:f=w480:T2)
        n176 = Select(t=w483, s=w478, f=w482) -> (s? t:f=w481:dbl)
        n177 = Not(x=w478) -> (.not. x?=w479:bool)
      }
      frame "Close Stabilizer" {
        # "Part of storage sequence"
        # "Hold pos while waiting for stabilizer\nto close"
        n178 = global read "Robot Global Data.vi" "Dashboard Packet"() -> (w503:T10)
        n179 = Unbundle By Name(w503) -> ("Elevator.Stabilizer Close Time"=w502:dbl)
        n180 = Greater Or Equal?(x=w504, y=w502) -> (x >= y?=w497:bool)
        n181 = Select(t=Elevator_State."Idle", s=w497, f=w501) -> (s? t:f=w494:T2)
      }
      frame "HP Load Unfinish" {
        n182 = global read "Robot Global Data.vi" "Dashboard Packet"() -> (w512:T10)
        n183 = Unbundle By Name(w512) -> ("Elevator.Stabilizer Open Time"=w511:dbl)
        n184 = Greater Or Equal?(x=w508, y=w511) -> (x >= y?=w510:bool)
        n185 = Select(t=Elevator_State."HP Load Wait" ("f"), s=w510, f=w507) -> (s? t:f=w505:T2)
      }
      frame "HP Load Score" {
        w520 = FALSE
        n186 = Unbundle By Name(w522) -> ("HP Drag Score"=w521:dbl)
        n187 = case shown="\"Idle\", Default" w518 {
          tunnel: [w523 Elevator_State."Idle" ("f")] -> w517
          tunnel: w516 -> [w523 _]
          frame "Idle", Default {
          }
          frame "Load 1".."Load 3", "Load Trashcan" {
          }
        }
      }
      frame "HP Load Finish" {
        w527 = TRUE ("Boolean")
        # "Hold position, finish is complete"
        n188 = case shown="\"Load 3\"" w530 {
          tunnel: [w531 Elevator_State."HP Load Unfinish" ("f") Elevator_State."HP Load Score" ("f") Elevator_State."HP Load Score" ("f")] -> w529
          tunnel: w528 -> [w531 _ _ _]
          frame "Idle", Default {
          }
          frame "Load 1" {
          }
          frame "Load 3" {
            # "just because..."
          }
          frame "Drop Stack" {
          }
        }
      }
      frame "HP Goto Finish Down" {
        # "Can will be high enough to stabilize at lowest possible elevator height\n(when dragging 2, IE \"Drag Finish\"), so go there"
        n189 = Unbundle By Name(w545) -> ("HP Drag Finish"=w544:dbl)
        n190 = case shown="\"Load 2\"" w541 {
          tunnel: w540 -> [w546 _]
          tunnel: [w546 Elevator_State."HP Load Finish" ("f")] -> w538
          frame "Idle", Default {
          }
          frame "Load 2" {
            # "Override in case of elevator stickiness"
          }
        }
        n191 = Select(t=Elevator_State."HP Load Finish" ("f"), s=w539, f=w538) -> (s? t:f=w536:T2)
      }
      frame "HP Goto Finish Up" {
        # "Lift the elavator until finger height (can height) is OK like we do\nfor can storage"
        n192 = global read "Robot Global Data.vi" "Dashboard Packet"() -> (w552:T10)
        n193 = Unbundle By Name(w552) -> ("Elevator.Finger Stop Store"=w551:dbl)
        n194 = global read "Robot Global Data.vi" "Dashboard Packet"() -> (w564:T10)
        n195 = Unbundle By Name(w564) -> ("Elevator.Finger Store"=w563:dbl)
        n196 = Unbundle By Name(w567) -> ("Store can max"=w566:dbl)
        n197 = case shown="\"Load 2\"" w557 {
          tunnel: w556 -> [w568 _]
          tunnel: [w568 Elevator_State."HP Load Finish" ("f")] -> w555
          frame "Idle", Default {
          }
          frame "Load 2" {
            # "Override for elevator stickiness"
          }
        }
        n198 = Greater Or Equal?(x=w553, y=w563) -> (x >= y?=w562:bool)
        n199 = Greater Or Equal?(x=w553, y=w551) -> (x >= y?=w550:bool)
        n200 = Or(x=w561, y=w562) -> (x .or. y?=w558:bool)
        n201 = Select(t=FALSE, s=w550, f=w554) -> (s? t:f=w548:bool)
        n202 = Select(t=Elevator_State."HP Load Finish" ("f"), s=w558, f=w555) -> (s? t:f=w559:T2)
      }
      frame "Full" {
        n203 = case shown="\"Drop Stack\"" w572 {
          tunnel: [w578 Elevator_State."Idle" ("f") Elevator_State."Drop Stack" ("f")] -> w571
          tunnel: w570 -> [w578 _ _]
          frame "Idle" {
          }
          frame "Load 1", Default {
          }
          frame "Drop Stack" {
          }
        }
        n204 = Unbundle By Name(w577) -> ("Full"=w576:dbl)
      }
    }
    "Trashcan Delta" <- w41
    "Tote Delta" <- w11
    n205 = Unbundle By Name("Command") -> ("Store Trashcan?"=w27:bool, "HP Load"=w26:bool, "Manual Eject Piston"=w23:bool)
    n206 = Or(x=w23, y=w25) -> (x .or. y?=w24:bool)
    n207 = Bundle By Name(cluster=T1 {"Target Out"=0.0, "Storing Trashcan?"=FALSE, "State"=enum."Idle", "In Range"=FALSE, "Store Can Command"=FALSE, "HP Load"=FALSE} ("Auto Elevator Indicators"), "Store Can Command"=w27, "HP Load"=w26, "In Range"=w32, "State"=w8, "Target Out"=w18, "Storing Trashcan?"=w14) -> (→"Auto Elevator Indicators":T1)
    n208 = Bundle By Name(cluster=T8 {"Ejector Piston"=FALSE, "Finger"=FALSE, "Stabilizer"=FALSE, "Position Out"=0.0} ("Elevator Actuators Out"), "Ejector Piston"=w24, "Finger"=w21, "Stabilizer"=w20, "Position Out"=w18) -> (→"Elevator Actuators Out":T8)
  }
  "Clear Stack Count" <- w1
